vi "DUAL GAUGE-RW Calibration factor.vi"(7 "W/R":bool, 8 "Fehler (Eingang)":errorcluster, 9 "Set Calibration factor2":dbl=1.0 min=0.1 max=9.999 step=0.001 format="%.3f", 10 "Set Calibration factor1":dbl=1.0 min=0.1 max=9.999 step=0.001 format="%.3f", 11 "Referenz in":refnum<visa-resource-name>) -> (0 "Cluster (Ausgang)":errorcluster, 1 "Get Calibration factor 2":dbl=0.000753 format="%.3f", 2 "Get Calibration factor 1":dbl=0.000753 format="%.3f", 3 "Referenz out":refnum<visa-resource-name>)   [LabVIEW 2017, in "Dual Gauge.lvlib"]
uses:
  <userlib>/Dual Gauge/Dual Gauge.lvlib
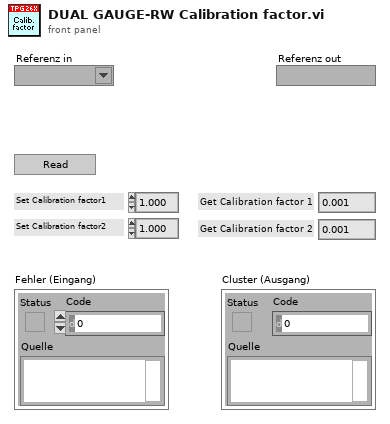
[diagram p1: front panel]
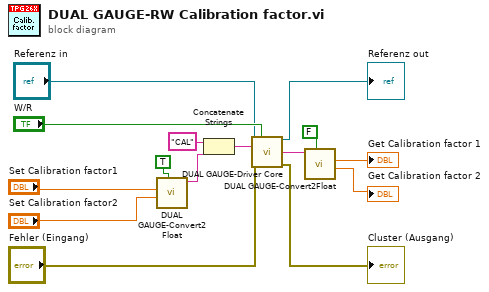
[diagram p0: block diagram]
diagram:
  n1 = call <userlib>:"DUAL GAUGE-Convert2Float.vi"("W/R [W: Int in; Str out ]"=TRUE, "Eng2 in"="Set Calibration factor2", "Eng1 in"="Set Calibration factor1") -> ("String out"=w8:string)  [unwired: 6 in, 2 out]
  n2 = Concatenate Strings("CAL", w8) -> (w5:string)
  n3 = call <userlib>:"DUAL GAUGE-Driver Core.vi"("Referenz in"="Referenz in", "Write/Read"="W/R", "Command"=w5, "Fehler (Eingang)"="Fehler (Eingang)") -> ("Referenz out"=→"Referenz out":refnum<visa-resource-name>, "String Out"=w6:string, "Cluster (Ausgang)"=→"Cluster (Ausgang)":errorcluster)  [unwired: 9 in]
  n4 = call <userlib>:"DUAL GAUGE-Convert2Float.vi"("W/R [W: Int in; Str out ]"=FALSE, "String in"=w6) -> ("Eng2 out"=→"Get Calibration factor 2":dbl, "Eng1 out"=→"Get Calibration factor 1":dbl)  [unwired: 7 in, 1 out]
